vi "Execute SQL.vi"(7 "Use SAVEPOINT":bool, 8 "error in (no error)":errorcluster, 10 "SQL":string, 11 "SQLite Connection in":refnum<class "Connection.lvclass">) -> (0 "error out":errorcluster, 1 "Column Names":string[](array[string]), 2 "Result Set":string[][](table) caption="Result Set (from first statement with results)", 3 "SQLite Connection out":refnum<class "Connection.lvclass">)   [LabVIEW 2011, in "SQLite.lvlib" / "Connection.lvclass"]
doc: "Executes an SQL script containing one or more SQL statements. If one of the statements returns results, these are returned as a 2D array of strings. Results from additional statements will not be returned; use this VI multiple times to get results of multiple statements."
uses:
  Connection.lvclass
  SQL Statement/SQL Statement.lvclass/SQL Statement.ctl
  SQL Statement/Get Column Count.vi
  SQL Statement/Write Next Column.vi
  SQL Statement/Get Column Name.vi
  SQL Statement/Step.vi
  SQL Statement/Error Message.vi
  SQL Statement/SQL Statement.lvclass
  SQLite.lvlib
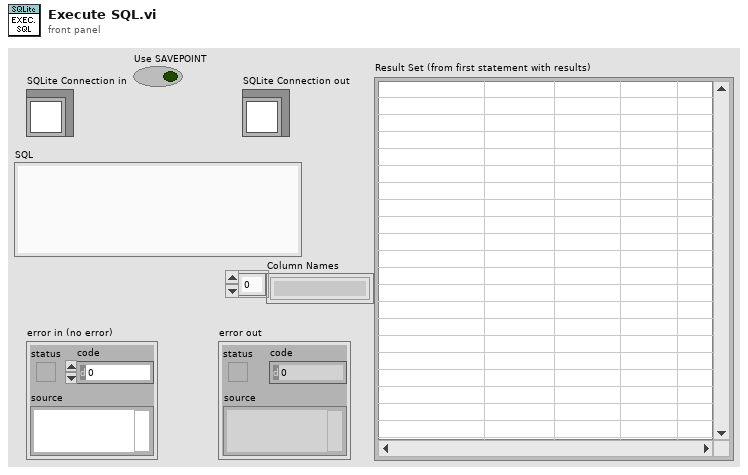
[diagram p1: front panel]
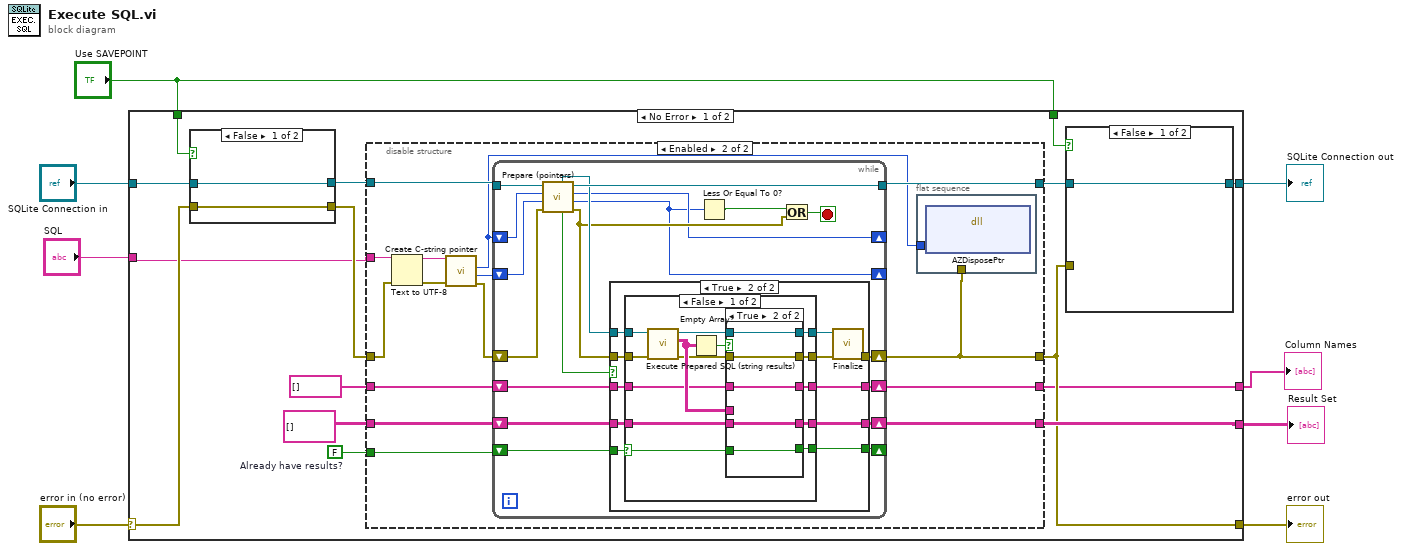
[diagram p0: block diagram]
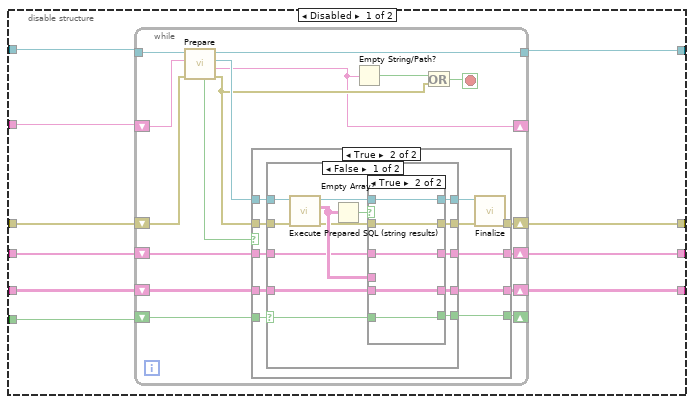
[diagram p2: hidden frame]
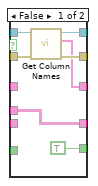
[diagram p4: hidden frame]
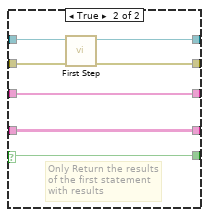
[diagram p5: hidden frame]
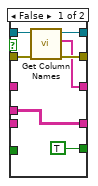
[diagram p7: hidden frame]
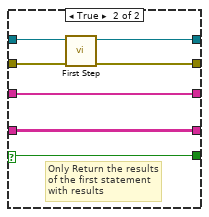
[diagram p8: hidden frame]
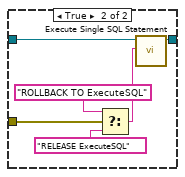
[diagram p9: hidden frame]
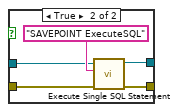
[diagram p10: hidden frame]
diagram:
  n1 = case shown="No Error" "error in (no error)" {
    selector: "error in (no error)" -> [w15 w197]
    tunnel: [w19 w197] -> w7
    tunnel: [w20 w196] -> w5
    tunnel: "SQLite Connection in" -> [w17 w196]
    tunnel: "SQL" -> [w9 _]
    tunnel: [w23 _] -> w3
    tunnel: "Use SAVEPOINT" -> [w13 _]
    tunnel: "Use SAVEPOINT" -> [w12 _]
    tunnel: [w10 _] -> w1
    frame No Error {
      w21 = FALSE  # Already have results?
      n2 = case shown="False" w13 {
        tunnel: w17 -> [w190 w194]
        tunnel: [w190 w193] -> w16
        tunnel: w15 -> [w189 w192]
        tunnel: [w189 w191] -> w14
        frame False {
        }
        frame True {
          n3 = call "Execute Single SQL Statement.vi"("error in (no error)"=w192, "SQL statement"="SAVEPOINT ExecuteSQL" ("SQL"), "SQLite Connection in"=w194) -> ("error out"=w191:errorcluster, "SQLite Connection out"=w193:refnum<class "Connection.lvclass">)  [unwired: 7 in]
        }
      }
      n4 = disable-structure shown="Enabled" {
        disable-tunnel: w9 -> [w33 w104]
        disable-tunnel: [w32 w113] -> w23
        disable-tunnel: string[][] [] ("Result Set (Text)") -> [w31 w112]
        disable-tunnel: w21 -> [w30 w111]
        disable-tunnel: [w29 w101] -> w19
        disable-tunnel: [w28 w110] -> w18
        disable-tunnel: w16 -> [w27 w109]
        disable-tunnel: w14 -> [w26 w100]
        disable-tunnel: string[] [] ("Column Names") -> [w25 w108]
        disable-tunnel: [w24 w107] -> w10
        frame Disabled {
          n5 = while {
            tunnel: w27 -> [w50]
            tunnel: [w49] -> w28
            shift-right: [w34] -> _
            shift-left: w33 -> [w48]
            shift-right: [w44] -> w32
            shift-left: w31 -> [w42]
            shift-right: [w40] -> _
            shift-left: w30 -> [w41]
            shift-right: [w46] -> w29
            shift-left: w26 -> [w47]
            shift-right: [w37] -> w24
            shift-left: w25 -> [w36]
            stop <- w39 stop-if-true
            n6 = call "Prepare.vi"("error in (no error)"=w47, "SQL"=w48, "SQLite Connection in"=w50) -> ("error out"=w38:errorcluster, "Rest of SQL"=w34:string, "SQL Statement out"=w45:refnum<class "SQL Statement.lvclass">, "SQLite Connection out"=w49:refnum<class "Connection.lvclass">, "Valid Statement"=w35:bool)  [unwired: 4 in]
            n7 = case shown="True" w35 {
              tunnel: [w54 w65] -> w46
              tunnel: w45 -> [_ w64]
              tunnel: [w52 w61] -> w44
              tunnel: w42 -> [w52 w60]
              tunnel: w41 -> [w51 w59]
              tunnel: [w51 w58] -> w40
              tunnel: w38 -> [w54 w57]
              tunnel: [w53 w56] -> w37
              tunnel: w36 -> [w53 w55]
              frame False {
                # "Not a valid statement \n(could be just a comment or whitespace)"
              }
              frame True {
                n8 = case shown="False" w59 {
                  selector: w59 -> [w72 w93]
                  tunnel: w64 -> [w79 w98]
                  tunnel: w57 -> [w78 w97]
                  tunnel: [w70 w96] -> w63
                  tunnel: [w68 w95] -> w62
                  tunnel: [w75 w94] -> w61
                  tunnel: w60 -> [w76 w94]
                  tunnel: [w73 w93] -> w58
                  tunnel: [w67 w92] -> w56
                  tunnel: w55 -> [w66 w92]
                  frame False {
                    n9 = call "Execute Prepared SQL (string results).vi"("error in (no error)"=w78, "SQL Statement in"=w79) -> ("error out"=w69:errorcluster, "Result Set"=w74:string[][], "SQL Statement out"=w71:refnum<class "SQL Statement.lvclass">)  [unwired: 7 in]
                    n10 = Empty Array?(array=w74) -> (empty?=w77:bool)
                    n11 = case shown="True" w77 {
                      tunnel: w76 -> [_ w91]
                      tunnel: [w86 w91] -> w75
                      tunnel: w74 -> [w86 _]
                      tunnel: [TRUE w90] -> w73
                      tunnel: w72 -> [_ w90]
                      tunnel: w71 -> [w84 w89]
                      tunnel: [w83 w89] -> w70
                      tunnel: w69 -> [w82 w88]
                      tunnel: [w81 w88] -> w68
                      tunnel: [w80 w87] -> w67
                      tunnel: w66 -> [_ w87]
                      frame False {
                        n12 = call "Get Column Names.vi"("error in (no error)"=w82, "SQL Statement in"=w84) -> ("error out"=w81:errorcluster, "Column Names"=w80:string[], "SQL Statement out"=w83:refnum<class "SQL Statement.lvclass">)  [unwired: 7 in]
                      }
                      frame True {
                      }
                    }
                  }
                  frame True {
                    # "Only Return the results\nof the first statement\nwith results"
                    n13 = call "First Step.vi"("error in (no error)"=w97, "SQL Statement in"=w98) -> ("error out"=w95:errorcluster, "SQL Statement out"=w96:refnum<class "SQL Statement.lvclass">)  [unwired: 7 in, 1 out]
                  }
                }
                n14 = call "Finalize.vi"("error in (no error)"=w62, "SQL Statement in"=w63) -> ("error out"=w65:errorcluster)  [unwired: 9 in]
              }
            }
            n15 = Empty String/Path?(string/path=w34) -> (empty?=w43:bool)
            n16 = Or(x=w43, y=w38) -> (x .or. y?=w39:bool)
          }
        }
        frame Enabled {
          n17 = Text to UTF-8(8:w100, 11:w104) -> (0:w106:errorcluster, 3:w105:string)
          n18 = call "Create C-string pointer.vi"("error in (no error)"=w106, "string"=w105) -> ("error out"=w99:errorcluster, "size"=w103:i32, "C-string pointer"=w102:i64)  [unwired: 6 in, 1 out]
          n19 = while {
            tunnel: w109 -> [w133]
            tunnel: [w132] -> w110
            shift-right: [w117] -> _
            shift-left: w102 -> [w119]
            shift-right: [w128] -> w113
            shift-left: w112 -> [w127]
            shift-right: [w125] -> _
            shift-left: w111 -> [w126]
            shift-right: [w130] -> w101
            shift-left: w99 -> [w131]
            shift-right: [w122] -> w107
            shift-left: w108 -> [w121]
            shift-right: [w115] -> _
            shift-left: w103 -> [w118]
            stop <- w124 stop-if-true
            n20 = call "Prepare (pointers).vi"("error in (no error)"=w131, "Bytes in SQL"=w118, "SQL pointer"=w119, "SQLite Connection in"=w133) -> ("error out"=w123:errorcluster, "Remaining bytes"=w115:i32, "Remaining SQL Tail"=w117:i64, "SQLite Connection out"=w132:refnum<class "Connection.lvclass">, "Valid Statement"=w120:bool, "SQL Statement out"=w129:refnum<class "SQL Statement.lvclass">)  [unwired: 2 in]
            n21 = case shown="True" w120 {
              tunnel: [w137 w148] -> w130
              tunnel: w129 -> [_ w147]
              tunnel: [w135 w144] -> w128
              tunnel: w127 -> [w135 w143]
              tunnel: w126 -> [w134 w142]
              tunnel: [w134 w141] -> w125
              tunnel: w123 -> [w137 w140]
              tunnel: [w136 w139] -> w122
              tunnel: w121 -> [w136 w138]
              frame False {
                # "Not a valid statement \n(could be just a comment or whitespace)"
              }
              frame True {
                n22 = case shown="False" w142 {
                  selector: w142 -> [w155 w176]
                  tunnel: w147 -> [w162 w181]
                  tunnel: w140 -> [w161 w180]
                  tunnel: [w153 w179] -> w146
                  tunnel: [w151 w178] -> w145
                  tunnel: [w158 w177] -> w144
                  tunnel: w143 -> [w159 w177]
                  tunnel: [w156 w176] -> w141
                  tunnel: [w150 w175] -> w139
                  tunnel: w138 -> [w149 w175]
                  frame False {
                    n23 = call "Execute Prepared SQL (string results).vi"("error in (no error)"=w161, "SQL Statement in"=w162) -> ("error out"=w152:errorcluster, "Result Set"=w157:string[][], "SQL Statement out"=w154:refnum<class "SQL Statement.lvclass">)  [unwired: 7 in]
                    n24 = Empty Array?(array=w157) -> (empty?=w160:bool)
                    n25 = case shown="True" w160 {
                      tunnel: w159 -> [_ w174]
                      tunnel: [w169 w174] -> w158
                      tunnel: w157 -> [w169 _]
                      tunnel: [TRUE w173] -> w156
                      tunnel: w155 -> [_ w173]
                      tunnel: w154 -> [w167 w172]
                      tunnel: [w166 w172] -> w153
                      tunnel: w152 -> [w165 w171]
                      tunnel: [w164 w171] -> w151
                      tunnel: [w163 w170] -> w150
                      tunnel: w149 -> [_ w170]
                      frame False {
                        n26 = call "Get Column Names.vi"("error in (no error)"=w165, "SQL Statement in"=w167) -> ("error out"=w164:errorcluster, "Column Names"=w163:string[], "SQL Statement out"=w166:refnum<class "SQL Statement.lvclass">)  [unwired: 7 in]
                      }
                      frame True {
                      }
                    }
                  }
                  frame True {
                    # "Only Return the results\nof the first statement\nwith results"
                    n27 = call "First Step.vi"("error in (no error)"=w180, "SQL Statement in"=w181) -> ("error out"=w178:errorcluster, "SQL Statement out"=w179:refnum<class "SQL Statement.lvclass">)  [unwired: 7 in, 1 out]
                  }
                }
                n28 = call "Finalize.vi"("error in (no error)"=w145, "SQL Statement in"=w146) -> ("error out"=w148:errorcluster)  [unwired: 9 in]
              }
            }
            n29 = Less Or Equal To 0?(x=w115) -> (x <= 0?=w116:bool)
            n30 = Or(x=w116, y=w123) -> (x .or. y?=w124:bool)
          }
          n31 = flat-sequence {
            tunnel: w102 -> [w114]
            tunnel: w101 -> [_]
            frame #0 {
              n32 = dll-call lib="LabVIEW" fn="AZDisposePtr"("pointer"=w114) -> ()  [unwired: 5 in, 2 out]
            }
          }
        }
      }
      n33 = case shown="False" w12 {
        tunnel: [w182 w188] -> w20
        tunnel: w19 -> [_ w187]
        tunnel: w18 -> [w182 w183]
        frame False {
        }
        frame True {
          n34 = Select(t="ROLLBACK TO ExecuteSQL" ("SQL"), s=w187, f="RELEASE ExecuteSQL" ("SQL")) -> (s? t:f=w184:string)
          n35 = call "Execute Single SQL Statement.vi"("SQL statement"=w184, "SQLite Connection in"=w183) -> ("SQLite Connection out"=w188:refnum<class "Connection.lvclass">)  [unwired: 8 in, 1 out]
        }
      }
    }
    frame Error {
    }
  }
  "error out" <- w7
  "SQLite Connection out" <- w5
  "Result Set" <- w3
  "Column Names" <- w1
